vi "integer_division.vi"() -> ()   [LabVIEW 2019]
panel:
  out "floor(x/y)":i32
  out "output":i32
  in  "Input":i32
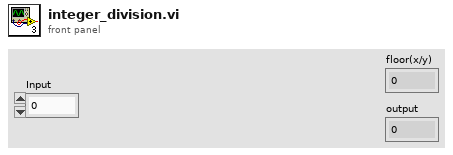
[diagram p1: front panel]
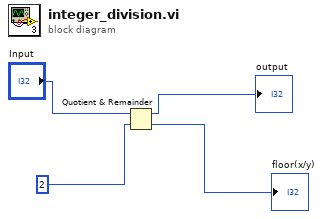
[diagram p0: block diagram]
diagram:
  n1 = Quotient & Remainder(x="Input", y=2 ("Input 2")) -> (x-y*floor(x/y)=→"output":i32, floor(x/y)=→"floor(x/y)":i32)
